vi "iikk.vi"() -> ()   [LabVIEW 2017]
uses:
  b161dac7-1d27-4718-bd9e-b9ae7e2b9074.vi
  global variable.vi
panel:
  out "추가된 배열":dbl[](array[numeric])
  out "Elapsed Time (s)":dbl caption="경과 시간(초)"
  out "첫 번째 부분배열":dbl[](array[numeric])
  in  "Gripper 각도":dbl
  in  "정지":bool
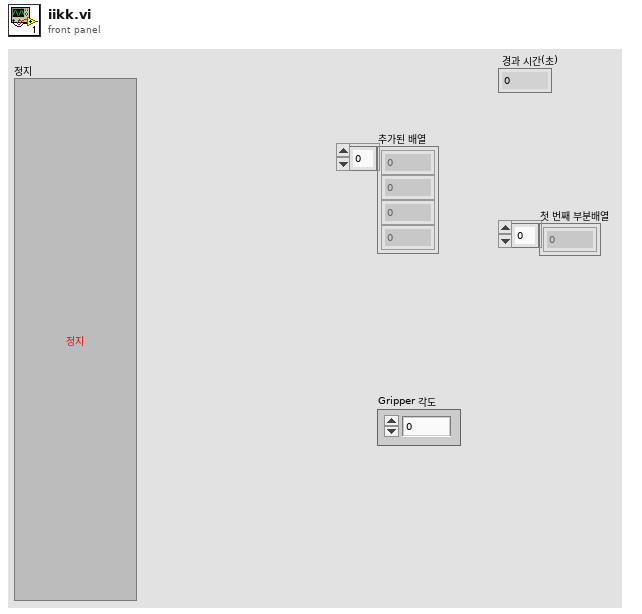
[diagram p1: front panel]
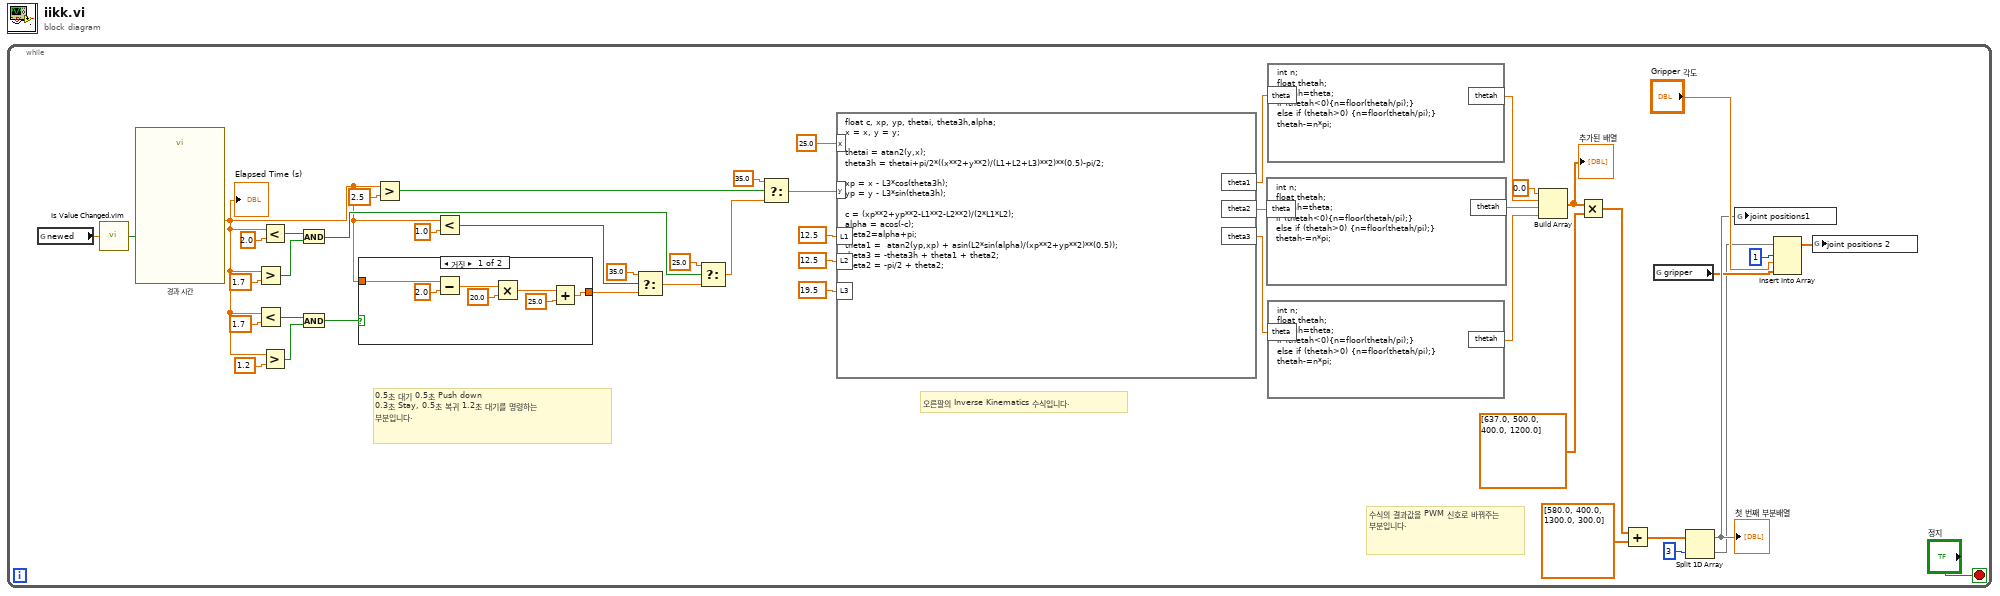
[diagram p0: block diagram]
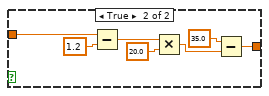
[diagram p2: hidden frame]
diagram:
  n1 = while {
    stop <- "정지" stop-if-true
    # "수식의 결과값을 PWM 신호로 바꿔주는\n부분입니다."
    # "오른팔의 Inverse Kinematics 수식입니다."
    # "0.5초 대기 0.5초 Push down\n0.3초 Stay, 0.5초 복귀 1.2초 대기를 명령하는\n부분입니다."
    n2 = global read "global variable.vi" "newed"() -> (w2:dbl)
    n3 = call "Is Value Changed.vim"("value"=w2) -> ("changed or first call?"=w1:bool)
    n4 = call "경과 시간"("Reset"=w1) -> ("Elapsed Time (s)"=w7:dbl)  [unwired: 11 in, 7 out]
    "Elapsed Time (s)" <- w7
    n5 = Greater?(x=w7, y=1.7 ("x")) -> (0:w16:bool)
    n6 = Less?(x=w7, y=1.7) -> (x < y?=w12:bool)
    n7 = Less?(x=w7, y=2.0) -> (x < y?=w14:bool)
    n8 = Greater?(x=w7, y=1.2) -> (0:w10:bool)
    n9 = And(x=w14, y=w16) -> (x .and. y?=w13:bool)
    n10 = And(x=w12, y=w10) -> (x .and. y?=w9:bool)
    n11 = case shown="거짓" w9 {
      tunnel: w7 -> [w51 w58]
      tunnel: [w52 w61] -> w4
      frame False {
        n12 = Subtract(x=w51, y=2.0) -> (x-y=w49:dbl)
        n13 = Multiply(x=w49, y=20.0) -> (x*y=w55:dbl)
        n14 = Add(x=w55, y=25.0) -> (x+y=w52:dbl)
      }
      frame True {
        n15 = Subtract(x=w58, y=1.2) -> (x-y=w56:dbl)
        n16 = Multiply(x=w56, y=20.0) -> (x*y=w59:dbl)
        n17 = Subtract(x=35.0, y=w59) -> (x-y=w61:dbl)
      }
    }
    n18 = Greater?(x=w7, y=2.5) -> (0:w30:bool)
    n19 = Less?(x=w7, y=1.0) -> (x < y?=w6:bool)
    n20 = Select(t=35.0, s=w6, f=w4) -> (s? t:f=w3:dbl)
    n21 = Select(t=25.0, s=w13, f=w3) -> (s? t:f=w18:dbl)
    n22 = Select(t=35.0, s=w30, f=w18) -> (s? t:f=w29:dbl)
    n23 = formula code="float c, xp, yp, thetai, theta3h,alpha;\nx = x, y = y;\n\nthetai = atan2(y,x);\ntheta3h = thetai+pi/2*((x**2+y**2)/(L1+L2+L3)**2)**(0.5)-pi/2;\n\nxp = x - L3*cos(theta3h);\nyp = y - L3*sin(theta3h);\n\nc = (xp**2+yp**2-L1**2-L2**2)/(2*L1*L2);\nalpha = acos(-c);\ntheta2=alpha+pi;\ntheta1 =  atan2(yp,xp) + asin(L2*sin(alpha)/(xp**2+yp**2)**(0.5));\ntheta3 = -theta3h + theta1 + theta2;\ntheta2 = -pi/2 + theta2;"("x"=25.0 ("입력 변수"), "y"=w29, "L1"=12.5 ("입력 변수"), "L2"=12.5 ("입력 변수"), "L3"=19.5 ("입력 변수")) -> ("theta1"=w27:dbl, "theta2"=w26:dbl, "theta3"=w25:dbl)
    n24 = formula code="int n;\nfloat thetah;\nthetah=theta;\nif (thetah<0){n=floor(thetah/pi);}\nelse if (thetah>0) {n=floor(thetah/pi);}\nthetah-=n*pi;"("theta"=w26) -> ("thetah"=w23:dbl)
    n25 = formula code="int n;\nfloat thetah;\nthetah=theta;\nif (thetah<0){n=floor(thetah/pi);}\nelse if (thetah>0) {n=floor(thetah/pi);}\nthetah-=n*pi;"("theta"=w27) -> ("thetah"=w24:dbl)
    n26 = formula code="int n;\nfloat thetah;\nthetah=theta;\nif (thetah<0){n=floor(thetah/pi);}\nelse if (thetah>0) {n=floor(thetah/pi);}\nthetah-=n*pi;"("theta"=w25) -> ("thetah"=w22:dbl)
    n27 = Build Array(0.0, w24, w23, w22) -> (w20:dbl[])
    "추가된 배열" <- w20
    n28 = Multiply(x=w20, y=dbl[] [637.0, 500.0, 400.0, 1200.0]) -> (x*y=w45:dbl[])
    n29 = Add(x=w45, y=dbl[] [580.0, 400.0, 1300.0, 300.0]) -> (x+y=w44:dbl[])
    n30 = global read "global variable.vi" "gripper"() -> (w32:dbl[])
    n31 = Split 1D Array(array=w44, index=3 ("인덱스")) -> (first subarray=w34:dbl[], second subarray=w21:dbl[])
    "첫 번째 부분배열" <- w34
    n32 = global write "global variable.vi" "joint positions1"(w34) -> ()
    n33 = Insert Into Array(array=w21, index=1 ("인덱스"), new element #1="Gripper 각도", new element #2=w32) -> (w33:dbl[])
    n34 = global write "global variable.vi" "joint positions 2"(w33) -> ()
  }
